vi "difficulty.vi"() -> ()   [LabVIEW 2025]
panel:
  out "Difficulty":u32
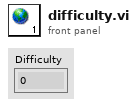
[diagram p1: front panel]
diagram:
